vi "getModeNRange.vi"(8 "error in (no error)":errorcluster, 11 "ElectrometerController in":refnum<class "ElectrometerController.lvclass">) -> (0 "error out":errorcluster, 1 "Input Range":dbl, 2 "Mode":T1, 3 "ElectrometerController out":refnum<class "ElectrometerController.lvclass">)   [LabVIEW 2016, in "ElectrometerController.lvclass"]
uses:
  ElectrometerController.lvclass
  Electrometer/Modes.ctl
  Electrometer/Electrometer.lvclass
  ElectrometerConfiguration/ElectrometerInternalConfiguration.lvclass
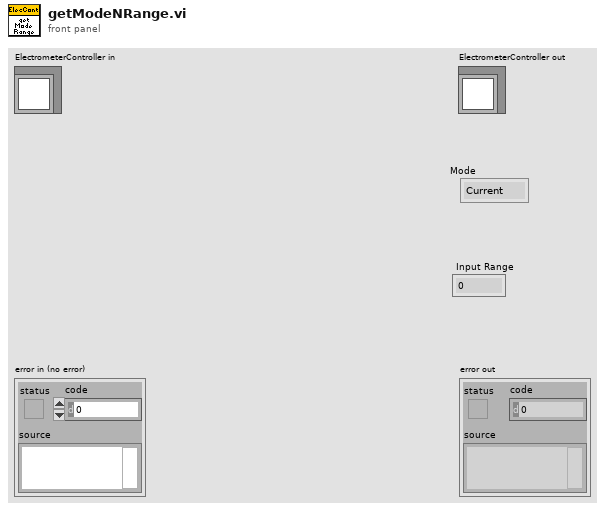
[diagram p1: front panel]
types:
  T1 = typedef "Electrometer.lvclass/Modes.ctl" = enum16{"Current", "Charge", "Voltage", "Resistance"}
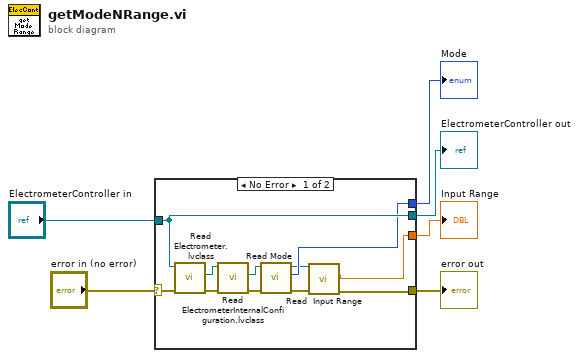
[diagram p0: block diagram]
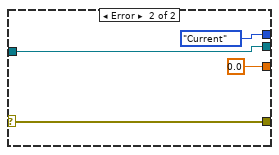
[diagram p2: hidden frame]
diagram:
  n1 = case shown="No Error" "error in (no error)" {
    selector: "error in (no error)" -> [w13 w21]
    tunnel: [w8 w21] -> w5
    tunnel: [w17 w20] -> w3
    tunnel: "ElectrometerController in" -> [w17 w20]
    tunnel: [w7 0.0 ("Input Range (Current)")] -> w2
    tunnel: [w11 Modes."Current" ("Measurement Function (0: Current)")] -> w1
    frame No Error {
      n2 = call-dynamic "Read Electrometer.lvclass.vi"("error in (no error)"=w13, "ElectrometerController in"=w17) -> ("error out"=w12:errorcluster, "Electrometer.lvclass"=w14:refnum<class "Electrometer.lvclass">)  [unwired: 7 in, 1 out]
      n3 = call-dynamic "Read ElectrometerInternalConfiguration.lvclass.vi"("error in (no error)"=w12, "Electrometer in"=w14) -> ("error out"=w16:errorcluster, "ElectrometerInternalConfiguration.lvclass"=w15:refnum<class "ElectrometerInternalConfiguration.lvclass">)  [unwired: 7 in, 1 out]
      n4 = call-dynamic "Read Mode.vi"("error in (no error)"=w16, "ElectrometerInternalConfiguration in"=w15) -> ("error out"=w9:errorcluster, "Measurement Function (0: Current)"=w11:T1, "ElectrometerInternalConfiguration out"=w10:refnum<class "ElectrometerInternalConfiguration.lvclass">)  [unwired: 7 in]
      n5 = call-dynamic "Read  Input Range .vi"("error in (no error)"=w9, "ElectrometerInternalConfiguration in"=w10) -> ("error out"=w8:errorcluster, "Input Range"=w7:dbl)  [unwired: 7 in, 1 out]
    }
    frame Error {
    }
  }
  "error out" <- w5
  "ElectrometerController out" <- w3
  "Input Range" <- w2
  "Mode" <- w1
